vi "PSD Meter.vi"(5 "PSD Config":T1 {"Averaging"."averaging mode" items=["No averaging", "RMS averaging", "Peak hold"]; "Averaging"."weighting mode" items=["Linear", "Exponential"]; "AR"."Method" items=["Forward-Backward", "Least-Squares", "Yule-Walker", "Burg-Lattice", "Geometric-Lattice"]; "Welch"."window info"."window" items=["None ", "Hanning", "Hamming", "Blackman-Harris", "Exact Blackman", "Blackman", "Flat Top", "4 Term B-Harris ", "7 Term B-Harris", "Low Sidelobe"]}, 6 "Reset":bool=TRUE, 7 "Set":T2 {"PSD Filter"."Forward Coefficients" format="%.4f"; "PSD Filter"."Reverse Coefficients" format="%.4f"}, 8 "error in (no error)":errorcluster, 11 "DATA IN":waveform(dbl)) -> (0 "error out":errorcluster, 3 "PSD Out":cluster{"f0":dbl, "df":dbl, "S(f)":dbl[]}[](array[cluster]))   [LabVIEW 2017, in "Processing.lvlib"]
uses:
  Processing.lvlib
  Filters.ctl
  PSD Setting.ctl
  <vilib>/Analysis/2dsp.llb/Decimate (single shot, DBL).vi
  <vilib>/Analysis/baseanly.llb/IIR Cascade Filter (DBL).vi
  <vilib>/addons/Time Series Analysis/Correlation and Spectral Analysis.llb/TSA Welch (Waveform).vi
  <vilib>/addons/Time Series Analysis/Correlation and Spectral Analysis.llb/TSA AR Spectrum (Waveform).vi
  <vilib>/Analysis/NI_AALBase.lvlib
  <vilib>/addons/_Advanced Signal Processing/NI_AdvSigProcTSA.lvlib
  <vilib>/Analysis/NI_AALPro.lvlib
panel:
  out "completed averages":u32
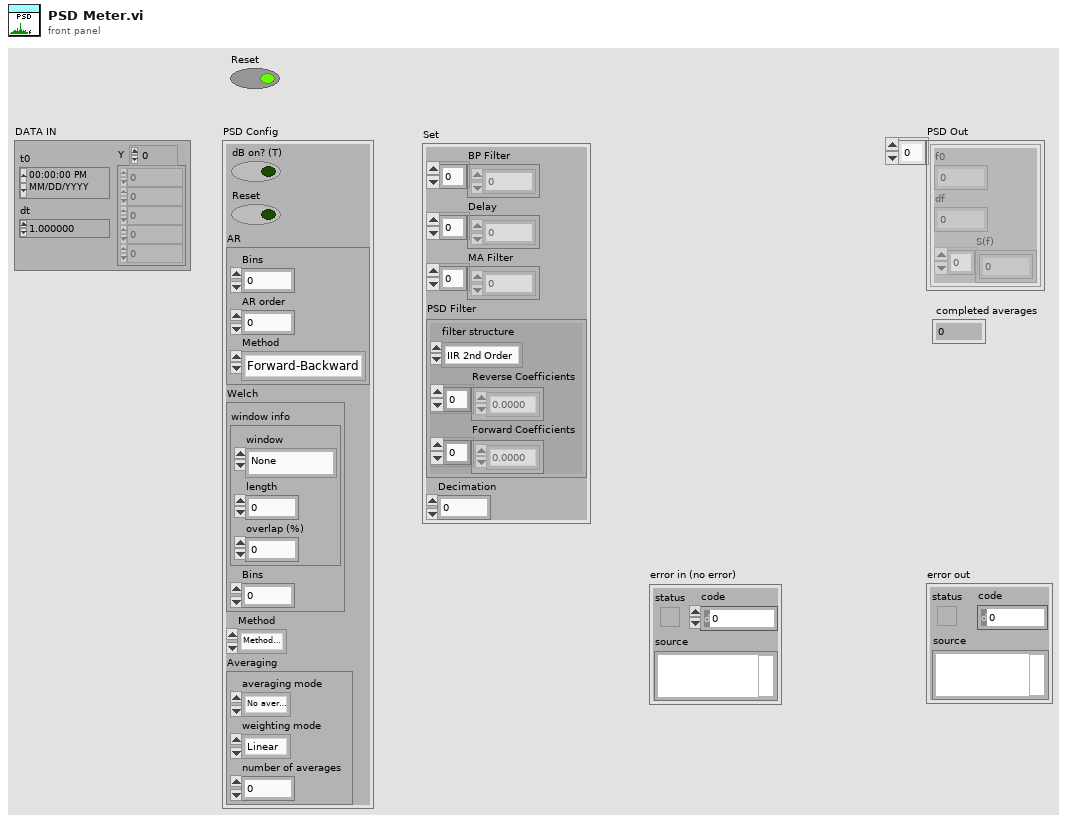
[diagram p1: front panel]
types:
  T1 = typedef "Processing.lvlib/PSD Setting.ctl" = cluster{"dB on? (T)":bool, "Reset":bool, "AR":cluster{"Bins":i32, "AR order":i32, "Method":u16}, "Welch":cluster{"window info":cluster{"window":u16, "length":i32, "overlap (%)":dbl}, "Bins":i32}, "Method":enum16{"Method Welch", "Method AR", "Both"}, "Averaging":cluster{"averaging mode":u16, "weighting mode":u16, "number of averages":u32}}
  T2 = typedef "Processing.lvlib/Filters.ctl" = cluster{"BP Filter":dbl[], "Delay":dbl[], "MA Filter":dbl[], "PSD Filter":cluster{"filter structure":enum32{"IIR 2nd Order", "IIR 4th Order"}, "Reverse Coefficients":dbl[], "Forward Coefficients":dbl[]}, "Decimation":i32}
  T3 = cluster{"filter structure":enum32{"IIR 2nd Order", "IIR 4th Order"}, "Reverse Coefficients":dbl[], "Forward Coefficients":dbl[]}
  T4 = cluster{"averaging mode":u16, "weighting mode":u16, "number of averages":u32}
  T5 = cluster{"window":u16, "length":i32, "overlap (%)":dbl}
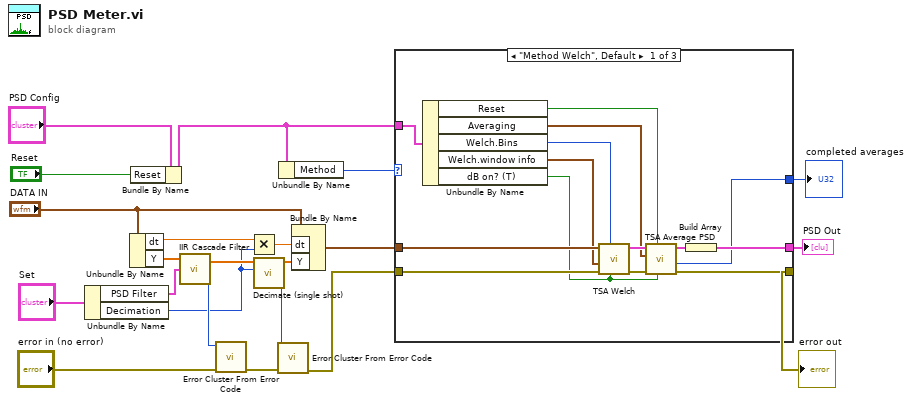
[diagram p0: block diagram]
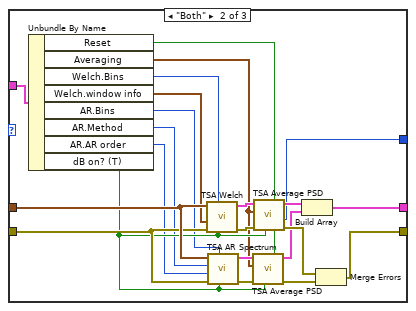
[diagram p2: hidden frame]
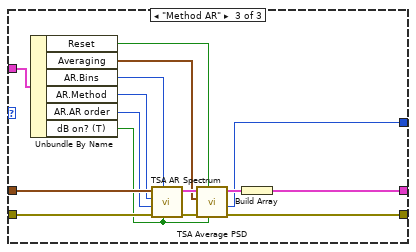
[diagram p3: hidden frame]
diagram:
  n1 = Unbundle By Name("Set") -> ("PSD Filter"=w13:T3, "Decimation"=w4:i32)
  n2 = Unbundle By Name("DATA IN") -> ("dt"=w5:dbl, "Y"=w15:dbl[])
  n3 = Bundle By Name(cluster="PSD Config", "Reset"="Reset") -> (w3:T1)
  n4 = call-poly <vilib>:"IIR Cascade Filter.vi"("IIR Filter Cluster"=w13, "X"=w15) -> ("error"=w16:i32, "Filtered X"=w12:dbl[])  [unwired: 1 in]
  n5 = call <vilib>:"Error Cluster From Error Code.vi"("error in (no error)"="error in (no error)", "error code (0)"=w16) -> ("error out"=w18:errorcluster)  [unwired: 7 in]
  n6 = Multiply(x=w5, y=w4) -> (x*y=w9:dbl)
  n7 = call-poly <vilib>:"Decimate (single shot).vi"("decimating factor"=w4, "X"=w12) -> ("error"=w19:i32, "Decimated Array"=w11:dbl[])  [unwired: 8 in]
  n8 = call <vilib>:"Error Cluster From Error Code.vi"("error in (no error)"=w18, "error code (0)"=w19) -> ("error out"=w20:errorcluster)  [unwired: 7 in]
  n9 = Unbundle By Name(w3) -> ("Method"=w21:enum16{"Method Welch", "Method AR", "Both"})
  n10 = Bundle By Name(cluster="DATA IN", "dt"=w9, "Y"=w11) -> (w17:waveform(dbl))
  n11 = case shown="\"Method Welch\", Default" w21 {
    tunnel: w17 -> [w30 w47 w73]
    tunnel: [w32 w52 w72] -> w8
    tunnel: w20 -> [w31 w46 w71]
    tunnel: w3 -> [w26 w58 w70]
    tunnel: [w33 w49 w61] -> w22
    tunnel: [w23 w37 w59] -> w1
    frame "Method Welch", Default {
      n12 = Unbundle By Name(w26) -> ("Reset"=w25:bool, "Averaging"=w29:T4, "Welch.Bins"=w28:i32, "Welch.window info"=w27:T5, "dB on? (T)"=w24:bool)
      n13 = call-poly <vilib>:"TSA Welch.vi"("dB on? (T)"=w24, "frequency bins"=w28, "error in (no error)"=w31, "window info"=w27, "Xt"=w30) -> ("error out"=w35:errorcluster, "PSD"=w36:cluster{"f0":dbl, "df":dbl, "S(f)":dbl[]})  [unwired: 4 in, 1 out]
      n14 = call <vilib>:"TSA Average PSD.vi"("dB on? (T)"=w24, "reset? (F)"=w25, "error in (no error)"=w35, "averaging parameters"=w29, "PSD"=w36) -> ("error out"=w32:errorcluster, "completed averages"=w23:u32, "PSD averaged"=w34:cluster{"f0":dbl, "df":dbl, "S(f)":dbl[]})  [unwired: 4 out]
      n15 = Build Array(w34) -> (w33:cluster{"f0":dbl, "df":dbl, "S(f)":dbl[]}[])
    }
    frame "Both" {
      n16 = Unbundle By Name(w58) -> ("Reset"=w45:bool, "Averaging"=w41:T4, "Welch.Bins"=w40:i32, "Welch.window info"=w39:T5, "AR.Bins"=w43:i32, "AR.Method"=w38:u16, "AR.AR order"=w42:i32, "dB on? (T)"=w44:bool)
      n17 = call-poly <vilib>:"TSA Welch.vi"("dB on? (T)"=w44, "frequency bins"=w40, "error in (no error)"=w46, "window info"=w39, "Xt"=w47) -> ("error out"=w56:errorcluster, "PSD"=w57:cluster{"f0":dbl, "df":dbl, "S(f)":dbl[]})  [unwired: 4 in, 1 out]
      n18 = call-poly <vilib>:"TSA AR Spectrum.vi"("dB on? (T)"=w44, "frequency bins"=w43, "error in (no error)"=w46, "AR order"=w42, "AR method"=w38, "Xt"=w47) -> ("error out"=w53:errorcluster, "PSD"=w54:cluster{"f0":dbl, "df":dbl, "S(f)":dbl[]})  [unwired: 4 out]
      n19 = call <vilib>:"TSA Average PSD.vi"("dB on? (T)"=w44, "reset? (F)"=w45, "error in (no error)"=w53, "averaging parameters"=w41, "PSD"=w54) -> ("error out"=w50:errorcluster, "PSD averaged"=w48:cluster{"f0":dbl, "df":dbl, "S(f)":dbl[]})  [unwired: 5 out]
      n20 = call <vilib>:"TSA Average PSD.vi"("dB on? (T)"=w44, "reset? (F)"=w45, "error in (no error)"=w56, "averaging parameters"=w41, "PSD"=w57) -> ("error out"=w51:errorcluster, "completed averages"=w37:u32, "PSD averaged"=w55:cluster{"f0":dbl, "df":dbl, "S(f)":dbl[]})  [unwired: 4 out]
      n21 = Build Array(w55, w48) -> (w49:cluster{"f0":dbl, "df":dbl, "S(f)":dbl[]}[])
      n22 = Merge Errors(w51, w50) -> (w52:errorcluster)
    }
    frame "Method AR" {
      n23 = Unbundle By Name(w70) -> ("Reset"=w63:bool, "Averaging"=w64:T4, "AR.Bins"=w65:i32, "AR.Method"=w66:u16, "AR.AR order"=w67:i32, "dB on? (T)"=w60:bool)
      n24 = call-poly <vilib>:"TSA AR Spectrum.vi"("dB on? (T)"=w60, "frequency bins"=w65, "error in (no error)"=w71, "AR order"=w67, "AR method"=w66, "Xt"=w73) -> ("error out"=w68:errorcluster, "PSD"=w69:cluster{"f0":dbl, "df":dbl, "S(f)":dbl[]})  [unwired: 4 out]
      n25 = call <vilib>:"TSA Average PSD.vi"("dB on? (T)"=w60, "reset? (F)"=w63, "error in (no error)"=w68, "averaging parameters"=w64, "PSD"=w69) -> ("error out"=w72:errorcluster, "completed averages"=w59:u32, "PSD averaged"=w62:cluster{"f0":dbl, "df":dbl, "S(f)":dbl[]})  [unwired: 4 out]
      n26 = Build Array(w62) -> (w61:cluster{"f0":dbl, "df":dbl, "S(f)":dbl[]}[])
    }
  }
  "error out" <- w8
  "PSD Out" <- w22
  "completed averages" <- w1
